vi "testRegCmdServersAandB.vi"(8 "error in (no error)":errorcluster) -> (0 "error out":errorcluster)   [LabVIEW 2018]
doc: "Test the getInstanceGen.vi in TCP/IP servers A and B."
uses:
  src/TcpServer/TcpServer.lvclass
  src/TcpServer/TcpServer.lvclass/TcpServer.ctl
  src/TcpServerCmd/TcpServerCmd.lvclass/TcpServerCmd.ctl
  <vilib>/addons/_JKI Toolkits/Caraya/classes/Assert/Assert Equal Value_Variant.vi
  src/TcpServerCmd/TcpServerCmd.lvclass
  <vilib>/addons/_JKI Toolkits/Caraya/classes/Test/Test.lvclass
  <vilib>/addons/_JKI Toolkits/Caraya/classes/Assert/Assert.lvclass
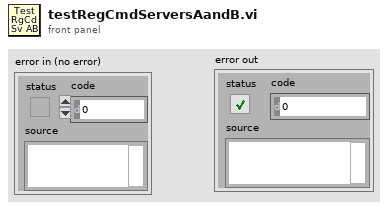
[diagram p1: front panel]
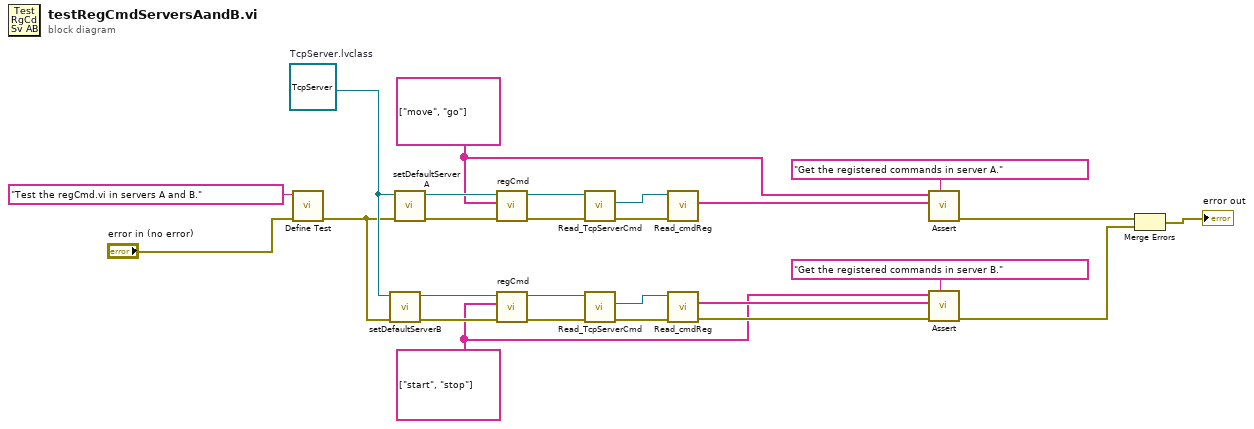
[diagram p0: block diagram]
diagram:
  w2 = string[] ["start", "stop"] ("registeredCommands")
  w5 = string[] ["move", "go"] ("registeredCommands")
  w23 = refnum<class "TcpServer.lvclass"> refnum  # TcpServer.lvclass
  n1 = call <vilib>:"Define Test.vi"("error in (no error)"="error in (no error)", "Label (VI Title)"="Test the regCmd.vi in servers A and B.") -> ("error out"=w22:errorcluster)  [unwired: 9 in]
  n2 = call "setDefaultServerB.vi"("error in (no error)"=w22, "TcpServer.lvclass"=w23) -> ("error out"=w10:errorcluster, "tcpServer out"=w9:refnum<class "TcpServer.lvclass">)  [unwired: 8 in]
  n3 = call "setDefaultServerA.vi"("error in (no error)"=w22, "TcpServer.lvclass"=w23) -> ("error out"=w16:errorcluster, "tcpServer out"=w15:refnum<class "TcpServer.lvclass">)  [unwired: 8 in]
  n4 = call "regCmd.vi"("error in (no error)"=w16, "cmdReg"=w5, "tcpServer in"=w15) -> ("error out"=w20:errorcluster, "tcpServer out"=w18:refnum<class "TcpServer.lvclass">)  [unwired: 7 in]
  n5 = call "regCmd.vi"("error in (no error)"=w10, "cmdReg"=w2, "tcpServer in"=w9) -> ("error out"=w11:errorcluster, "tcpServer out"=w13:refnum<class "TcpServer.lvclass">)  [unwired: 7 in]
  n6 = call "Read_TcpServerCmd.vi"("error in (no error)"=w20, "TcpServer in"=w18) -> ("error out"=w19:errorcluster, "TcpServerCmd.lvclass"=w17:refnum<class "TcpServerCmd.lvclass">)  [unwired: 7 in, 1 out]
  n7 = call "Read_TcpServerCmd.vi"("error in (no error)"=w11, "TcpServer in"=w13) -> ("error out"=w12:errorcluster, "TcpServerCmd.lvclass"=w14:refnum<class "TcpServerCmd.lvclass">)  [unwired: 7 in, 1 out]
  n8 = call "Read_cmdReg.vi"("error in (no error)"=w19, "TcpServerCmd in"=w17) -> ("cmdReg"=w6:string[])  [unwired: 7 in, 2 out]
  n9 = call "Read_cmdReg.vi"("error in (no error)"=w12, "TcpServerCmd in"=w14) -> ("error out"=w4:errorcluster, "cmdReg"=w3:string[])  [unwired: 7 in, 1 out]
  n10 = call-poly <vilib>:"Assert.vi"("Label"="Get the registered commands in server A.", "Y"=w6, "X"=w5) -> ("error out"=w24:errorcluster)  [unwired: 8 in]
  n11 = call-poly <vilib>:"Assert.vi"("Label"="Get the registered commands in server B.", "error in (no error)"=w4, "Y"=w3, "X"=w2) -> ("error out"=w1:errorcluster)  [unwired: 7 in]
  n12 = Merge Errors(w24, w1) -> (→"error out":errorcluster)
